vi "LateralController.vi"(0 "Xref":dbl[](array[numeric]), 1 "Yref":dbl[](array[numeric]), 2 "Psiref":dbl[](array[numeric]), 3 "X estimate":dbl, 4 "Y estimate":dbl, 5 "Psi estimate":dbl, 6 "error in (no error)":errorcluster, 7 "K1":dbl, 8 "closest_point":i8, 9 "K2":dbl, 10 "last_ids":dbl, 11 "e1_max":dbl) -> (14 "error out":errorcluster, 15 "idx":i8, 16 "last_ids_output":dbl, 19 "roll_ref":dbl)   [LabVIEW 2019]
uses:
  liblateral_controller-dummy.dll
  libpart_ref_trajectory-dummy.dll
panel:
  out "Psi ref size":i32
  out "X and Y ref size":i32
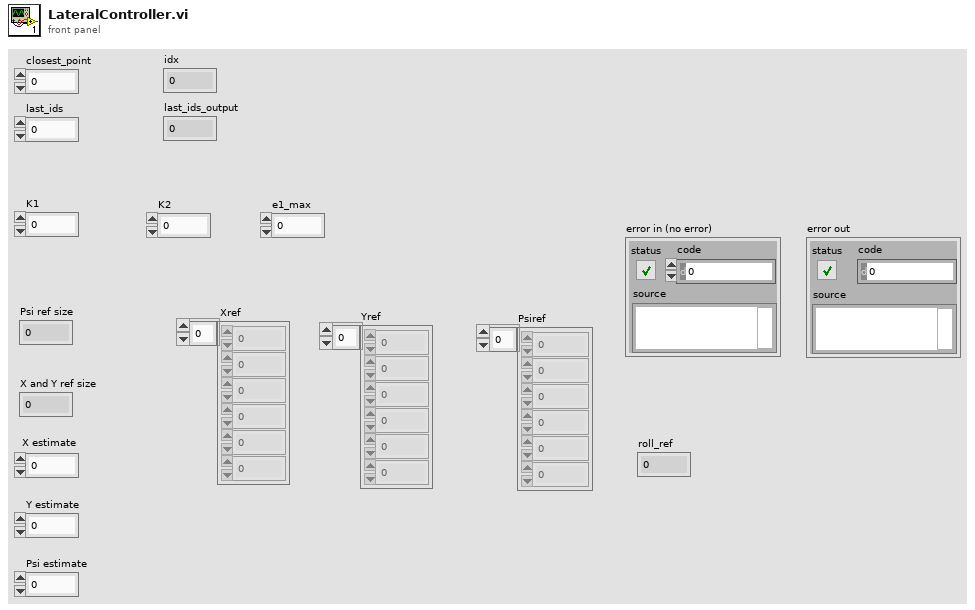
[diagram p1: front panel]
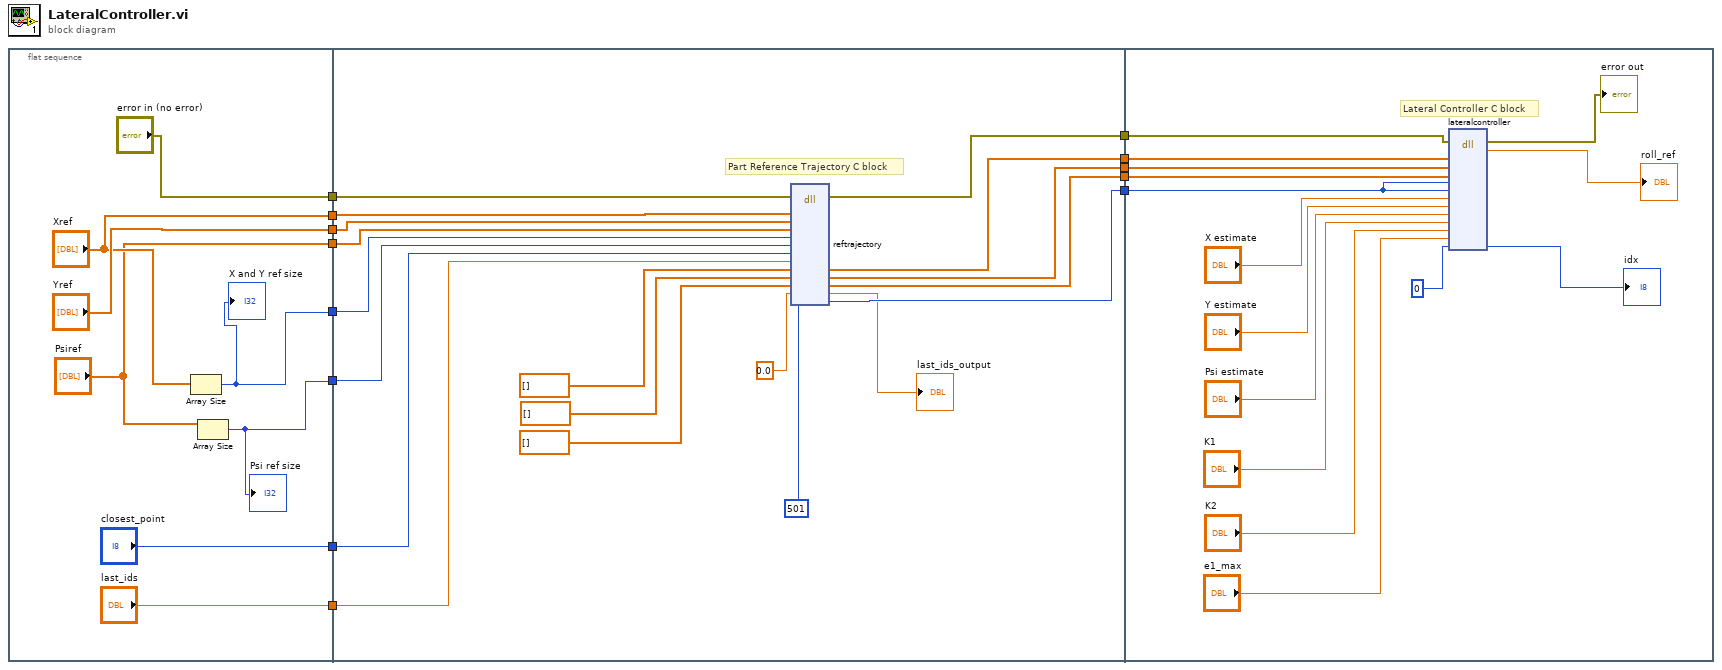
[diagram p0: block diagram]
diagram:
  n1 = flat-sequence {
    tunnel: ["error in (no error)"] -> w8
    tunnel: ["Xref"] -> w7
    tunnel: ["Yref"] -> w6
    tunnel: ["Psiref"] -> w5
    tunnel: [w18] -> w4
    tunnel: [w19] -> w3
    tunnel: ["last_ids"] -> w2
    tunnel: ["closest_point"] -> w1
    tunnel: [w30] -> w13
    tunnel: [w29] -> w12
    tunnel: [w28] -> w11
    tunnel: [w27] -> w10
    tunnel: [w25] -> w9
    tunnel: w8 -> [w40]
    tunnel: w7 -> [w39]
    tunnel: w6 -> [w38]
    tunnel: w5 -> [w33]
    tunnel: w4 -> [w32]
    tunnel: w3 -> [w31]
    tunnel: w2 -> [w23]
    tunnel: w1 -> [w22]
    tunnel: w13 -> [w48]
    tunnel: w12 -> [w47]
    tunnel: w11 -> [w46]
    tunnel: w10 -> [w45]
    tunnel: w9 -> [w44]
    frame #0 {
      n2 = Array Size(array="Xref") -> (size(s)=w18:i32)
      "X and Y ref size" <- w18
      n3 = Array Size(array="Psiref") -> (size(s)=w19:i32)
      "Psi ref size" <- w19
    }
    frame #1 {
      # "Part Reference Trajectory C block"
      n4 = dll-call lib="libpart_ref_trajectory-dummy.*" fn="reftrajectory"(error in=w40, "Xref"=w39, "Yref"=w38, "Psiref"=w33, "Xarraysize"=w32, "Psiarraysize"=w31, "closest_point"=w22, "last_ids"=w23, "local_Xref"=dbl[] [], "local_Yref"=dbl[] [], "local_Psiref"=dbl[] [], "last_ids_output"=0.0, "local_array_length"=501) -> (error out=w25:errorcluster, "local_Xref"=w29:dbl[], "local_Yref"=w28:dbl[], "local_Psiref"=w27:dbl[], "last_ids_output"=→"last_ids_output":dbl, "local_array_length"=w30:i32)  [unwired: 10 in, 1 out]
    }
    frame #2 {
      # "Lateral Controller C block"
      n5 = dll-call lib="liblateral_controller-dummy.*" fn="lateralcontroller"(error in=w44, "Xref"=w47, "Yref"=w46, "Psiref"=w45, "Xarraysize"=w48, "Psiarraysize"=w48, "Xest"="X estimate", "Yest"="Y estimate", "Psiest"="Psi estimate", "K1"="K1", "K2"="K2", "e1_max"="e1_max", "idx"=i8 0) -> (error out=→"error out":errorcluster, "roll_ref"=→"roll_ref":dbl, "idx"=→"idx":i8)  [unwired: 13 in, 1 out]
    }
  }
